vi "GetElementFromQueue.vi"(6 "error in (no error)":errorcluster, 9 "Queue in":refnum<queue>) -> (0 "error out":errorcluster, 1 "RxData":string, 2 "Consumer State":T1, 3 "queue out":refnum<queue>)   [LabVIEW 2019]
uses:
  ConsumerStates_ProjectBase.ctl
  QueueCluster_ProjectBase.ctl
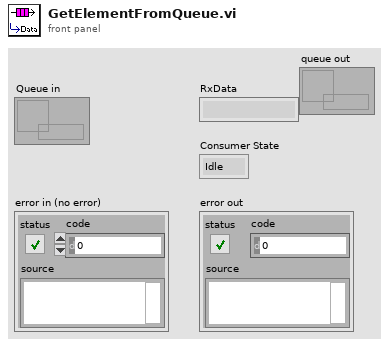
[diagram p1: front panel]
types:
  T1 = typedef "ConsumerStates_ProjectBase.ctl" = enum16{"Idle", "Generate TDMS", "Heating Sensor", "Catch Data", "Error"}
  T2 = typedef "QueueCluster_ProjectBase.ctl" = cluster{"error constant":errorcluster, "Consumer State":T1, "RxData":string}
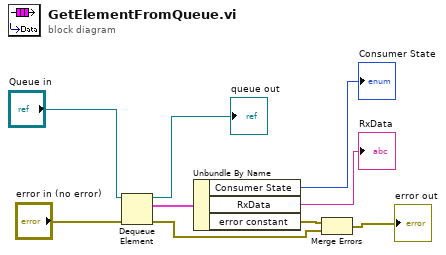
[diagram p0: block diagram]
diagram:
  n1 = Dequeue Element(queue="Queue in", error in (no error)="error in (no error)") -> (queue out=→"queue out":refnum<queue>, element=w7:T2, error out=w1:errorcluster)  [unwired: 1 in, 1 out]
  n2 = Unbundle By Name(w7) -> ("Consumer State"=→"Consumer State":T1, "RxData"=→"RxData":string, "error constant"=w2:errorcluster)
  n3 = Merge Errors(w2, w1) -> (→"error out":errorcluster)
